vi "niRFUtil FTW FIR Filter (real wfm).vi"(1 "Filter":T1 {"y" min=0 max=127 format="%.2f"; "dx" format="%^.2e"; "x0" format="%^.2e"}, 2 "Waveform In":T1 {"y" min=0 max=127 format="%.2f"; "dx" format="%^.2e"; "x0" format="%^.2e"}) -> (0 "Waveform Out":T1 {"y" min=0 max=127 format="%.2f"; "dx" format="%^.2e"; "x0" format="%^.2e"})   [LabVIEW 2015, in "niRFUtil.lvlib"]
doc: "(c) Copyright 2006, National Instruments, Inc. This VI may not be duplicated, sold, or distributed without written consent from National Instruments."
uses:
  niRFUtil.lvlib
  Includes/niRFUtil INC Real Waveform.ctl
  Includes/niRFUtil INC Real Array.ctl
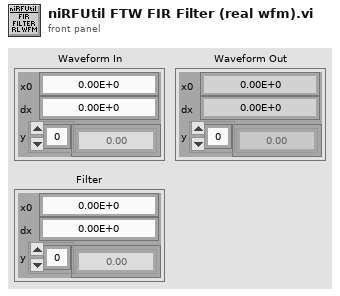
[diagram p1: front panel]
types:
  T1 = typedef "niRFUtil.lvlib/niRFUtil INC Real Waveform.ctl" = cluster{"x0":dbl, "dx":dbl, "y":T2}
  T2 = typedef "niRFUtil.lvlib/niRFUtil INC Real Array.ctl" = sgl[]
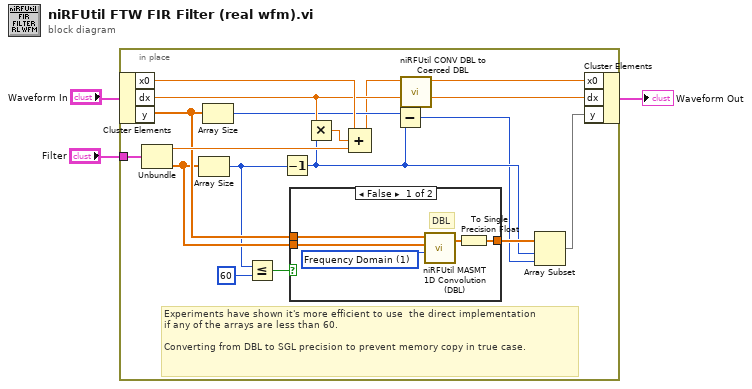
[diagram p0: block diagram]
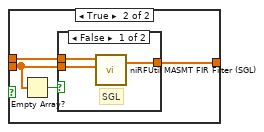
[diagram p2: hidden frame]
diagram:
  n1 = in-place {
    in-place-border: "Filter" -> [w18]
    # "Experiments have shown it's more efficient to use  the direct implementation\nif any of the arrays are less than 60. \n\nConverting from DBL to SGL precision to prevent memory copy in true case."
    n2 = in-place-cluster #1("Waveform In") -> ("x0"=w17:dbl, "dx"=w15:dbl, "y"=w16:T2)
    n3 = Unbundle(w18) -> ("x0"=w19:dbl, "y"=w9:T2)  [unwired: 1 out]
    n4 = Array Size(array=w9) -> (size(s)=w6:i32)
    n5 = Array Size(array=w16) -> (size(s)=w11:i32)
    n6 = Less Or Equal?(x=w6, y=60) -> (x <= y?=w8:bool)
    n7 = Decrement(x=w6) -> (x-1=w13:i32)
    n8 = case shown="False" w8 {
      tunnel: [w21 w29] -> w20
      tunnel: w16 -> [w25 w28]
      tunnel: w9 -> [w24 w27]
      frame False {
        w23 = 1 items=["Direct", "Frequency Domain"] ("algorithm")
        # "DBL"
        n9 = call "niRFUtil MASMT 1D Convolution (DBL).vi"("algorithm"=w23, "Y"=w24, "X"=w25) -> ("X * Y"=w22:dbl[])  [unwired: 7 in, 1 out]
        n10 = To Single Precision Float(number=w22) -> (single precision float=w21:sgl[])
      }
      frame True {
        n11 = Empty Array?(array=w27) -> (empty?=w26:bool)
        n12 = case shown="False" w26 {
          tunnel: [w32 _] -> w29
          tunnel: w28 -> [w31 _]
          tunnel: w27 -> [w30 _]
          frame False {
            # "SGL"
            n13 = call "niRFUtil MASMT FIR Filter (SGL).vi"("FIR Coefficients"=w30, "X"=w31) -> ("Filtered X"=w32:sgl[])  [unwired: 8 in, 1 out]
          }
          frame True {
          }
        }
      }
    }
    n14 = Multiply(x=w15, y=w13) -> (x*y=w14:dbl)
    n15 = Compound Arithmetic op=ADD(w17, w14, w19) -> (w5:dbl)
    n16 = Subtract(x=w11, y=w13) -> (x-y=w12:i32)
    n17 = call "niRFUtil CONV DBL to Coerced DBL.vi"("Numeric In (DBL)"=w5) -> ("Coerced Numeric Out (DBL)"=w4:dbl)  [unwired: 10 in]
    n18 = Array Subset(array=w20, index=w13, length=w12) -> (w10:sgl[])
    n19 = in-place-cluster #1("x0"=w4, "dx"=w15, "y"=w10) -> (→"Waveform Out":T1)
  }
